vi "CreateLogFile.vi"(8 "ErrorIn":errorcluster, 10 "TestName":string, 11 "LogFolder":path) -> (0 "ErrorOut":errorcluster, 3 "LogFile":path)   [LabVIEW 2018]
doc: "Create a new log file at the specified path. Generally, this is called once at the start of a test to create a file and write a header. Other VIs are used within the application to append the log file with test measurements.\n\nCopyright © 2011 Epimedia, Inc. All Rights Reserved.\n\nThe Epimedia Application Library is Copyright © 2009-2011 Epimedia, Inc. \nAll Rights Reserved. Used under license."
panel:
  # "Copyright © 2011 Epimedia, Inc. All Rights Reserved.\n\nThe Epimedia Application Library is Copyright © 2009-2011 Epimedia, Inc. \nAll Rights Reserved. Used under license."
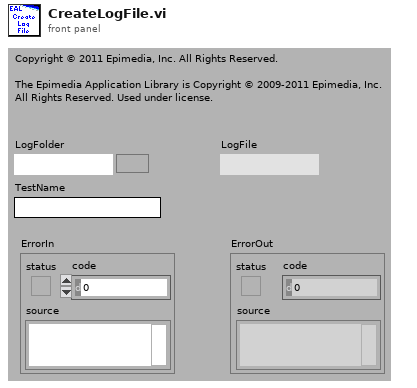
[diagram p1: front panel]
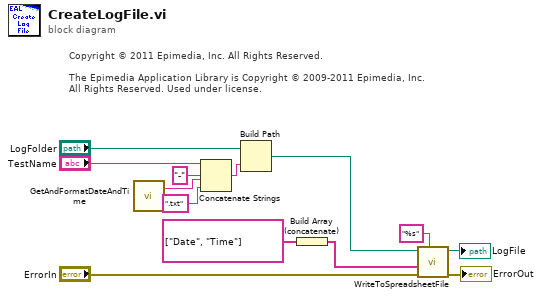
[diagram p0: block diagram]
diagram:
  # "Copyright © 2011 Epimedia, Inc. All Rights Reserved.\n\nThe Epimedia Application Library is Copyright © 2009-2011 Epimedia, Inc. \nAll Rights Reserved. Used under license."
  n1 = call "GetAndFormatDateAndTime.vi"() -> ("Date&Time"=w8:string)  [unwired: 3 in]
  n2 = Concatenate Strings("TestName", "-" ("string"), w8, ".txt" ("string")) -> (w13:string)
  n3 = Build Path(base path="LogFolder", name or relative path=w13) -> (appended path=w3:path)
  n4 = Build Array (concatenate)(string[] ["Date", "Time"]) -> (w6:string[])
  n5 = call "WriteToSpreadsheetFile.vi"("Prompt"="%s" ("format (%s)"), "ErrorIn"="ErrorIn", "1D-Data"=w6, "FilePath(DialogIfEmpty)"=w3) -> ("ErrorOut"=→"ErrorOut":errorcluster, "NewFilePath"=→"LogFile":path)  [unwired: 4 in, 2 out]
